vi "HandleCoincidenceData.vi"(4 "Added time":refnum<vi>, 6 "Seconds indicator":refnum<vi>, 7 "hit charts refnum cluster":T2, 8 "error in (no error)":errorcluster, 9 "coinc table":refnum<vi>, 10 "Seconds between updates":i32, 11 "Cluster":T3) -> (0 "error out":errorcluster)   [LabVIEW 2016]
uses:
  Typedefs/Coincidence histogram cluster refnum.ctl
  Typedefs/Hit chart cluster refnum.ctl
  Typedefs/Primary channel coincidence hunt.ctl
  Typedefs/Coincidence.ctl
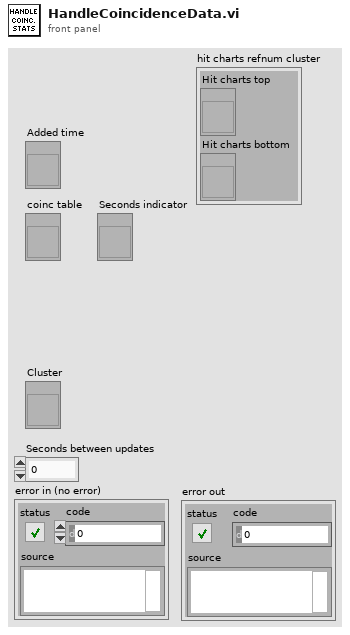
[diagram p1: front panel]
types:
  T1 = typedef "Hit chart cluster refnum.ctl" = refnum<vi>
  T2 = cluster{"Hit charts top":T1, "Hit charts bottom":T1}
  T3 = typedef "Coincidence histogram cluster refnum.ctl" = refnum<vi>
  T4 = typedef "Coincidence.ctl" = cluster{"Primary ID":i8, "Muon hit time":u64, "Secondary ID":i8, "DeltaT":i32}
  T5 = cluster{"Simultaneus muon tracks":cluster{"Top coinc":T4, "Bottom coinc":T4}[]}[]
  T6 = typedef "Primary channel coincidence hunt.ctl" = cluster{"Coincidences":T4[], "Secondary hits sorted":cluster{"ID":i8, "Non-coinc":u64[], "Coinc":u64[]}[], "Primary hits sorted":cluster{"ID":i8, "Non-coinc":u64[], "Coinc":u64[]}[]}
  T7 = cluster{"ID":i8, "Non-coinc":u64[], "Coinc":u64[]}[]
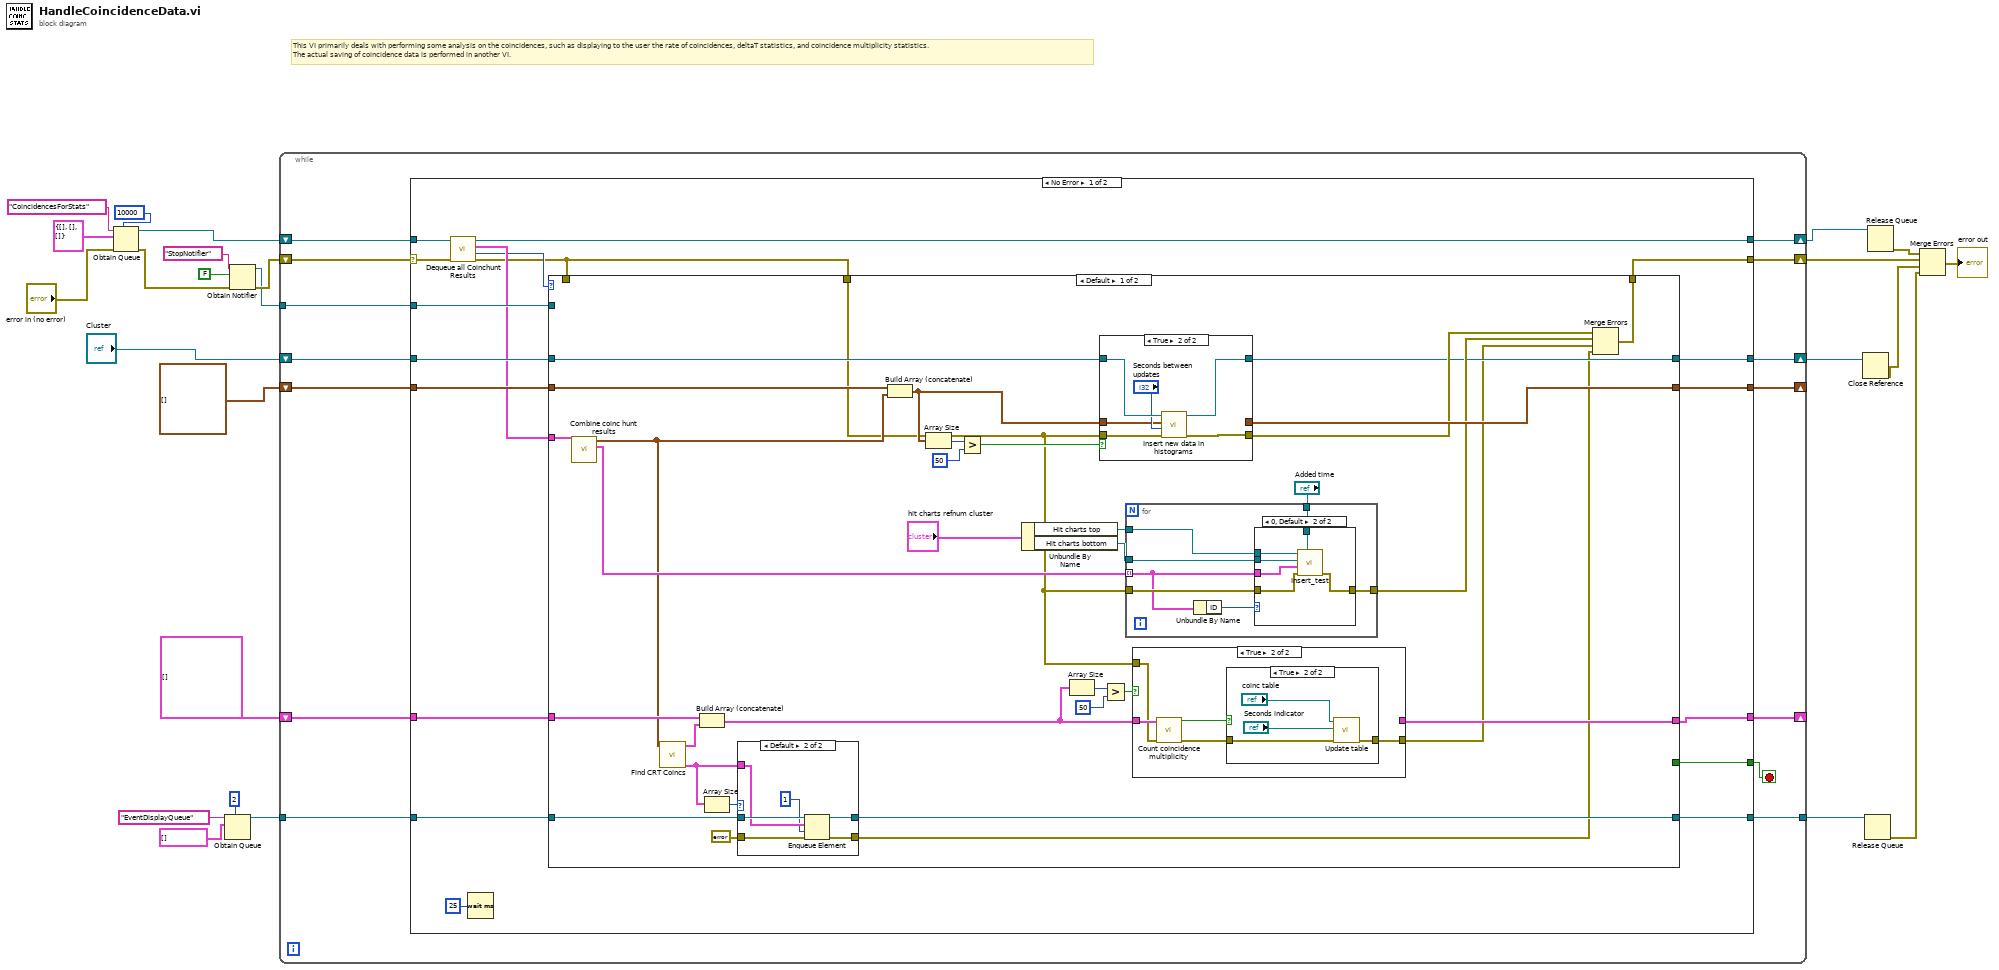
[diagram p0: block diagram]
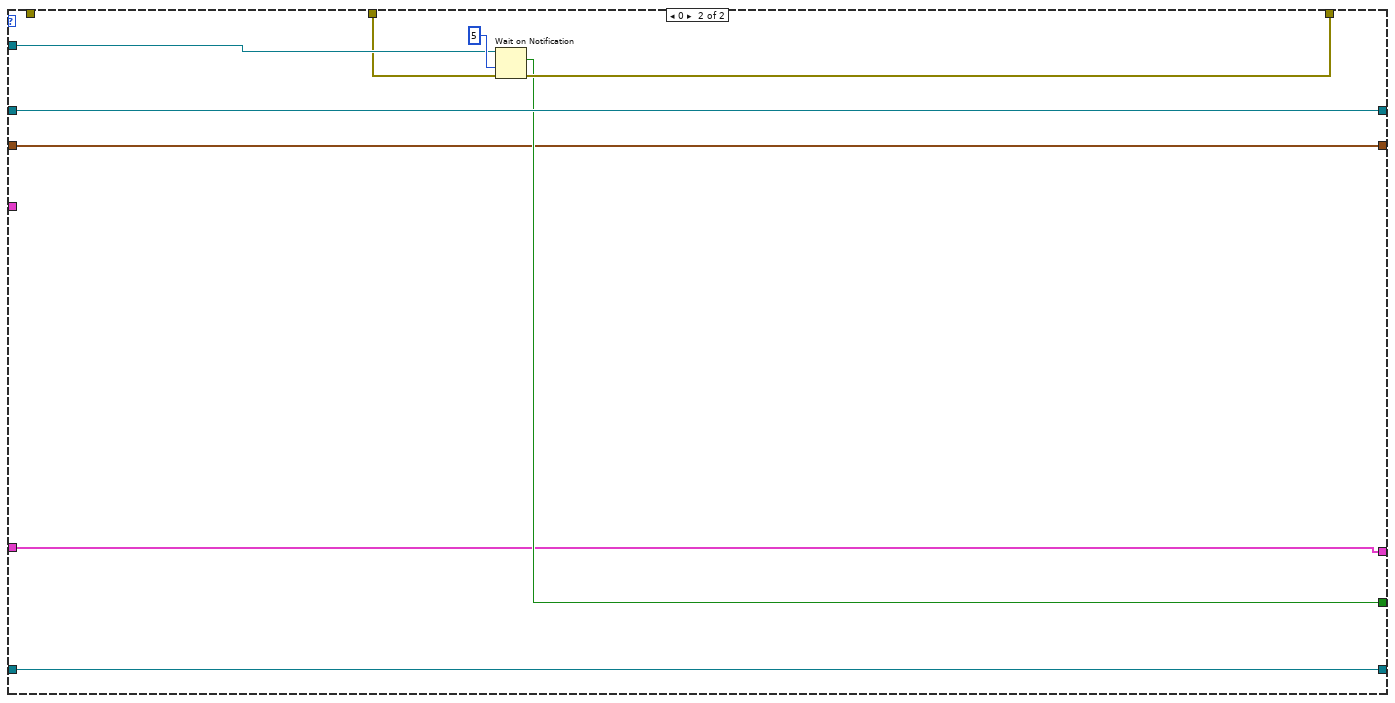
[diagram p7: hidden frame]
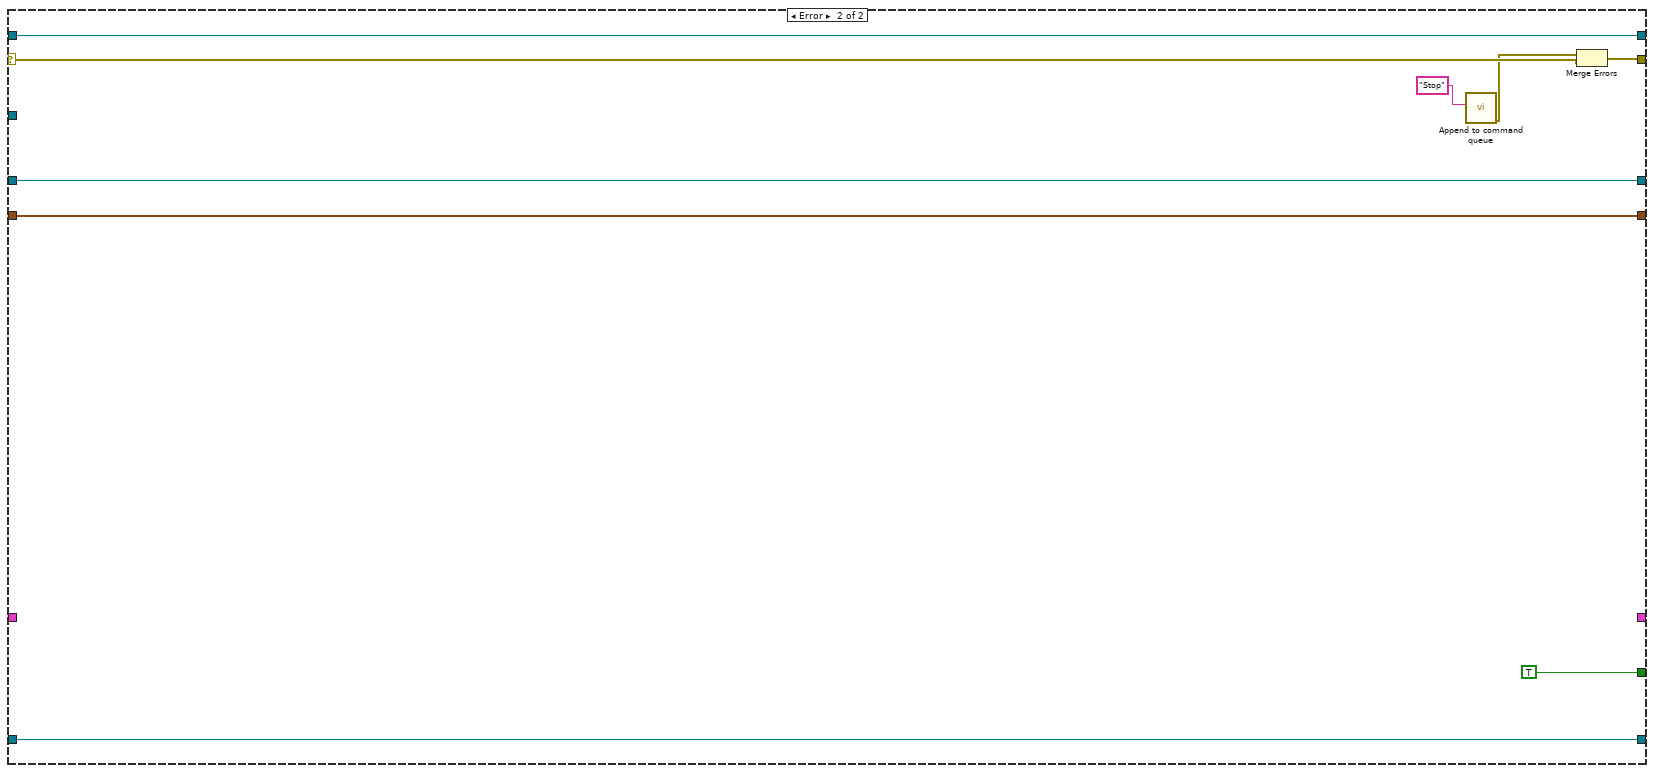
[diagram p8: hidden frame]
diagram:
  # "This VI primarily deals with performing some analysis on the coincidences, such as displaying to the user the rate of coincidences, deltaT statistics, and coincidence multiplicity statistics.\nThe actual saving of coincidence data is performed in another VI."
  n1 = Obtain Queue(max queue size (-1, unlimited)=10000, name (unnamed)="CoincidencesForStats", element data type=T6 {"Coincidences"=[], "Secondary hits sorted"=[], "Primary hits sorted"=[]} ("Planar coincidence hunt result"), error in (no error)="error in (no error)") -> (queue out=w24:refnum<queue>, error out=w17:errorcluster)  [unwired: 1 in, 1 out]
  n2 = Obtain Queue(max queue size (-1, unlimited)=2, name (unnamed)="EventDisplayQueue", element data type=T5 [] ("Good tracks")) -> (queue out=w4:refnum<queue>)  [unwired: 2 in, 2 out]
  n3 = Obtain Notifier(name (unnamed)="StopNotifier", notification data type=FALSE, error in (no error)=w17) -> (notifier out=w15:refnum<notifier>, error out=w16:errorcluster)  [unwired: 1 in, 1 out]
  n4 = while {
    shift-right: [w37] -> w14
    shift-left: w16 -> [w33]
    shift-right: [w38] -> w25
    shift-left: w24 -> [w39]
    shift-right: [w36] -> w11
    shift-left: "Cluster" -> [w32]
    tunnel: w15 -> [w34]
    shift-right: [w30] -> _
    shift-left: T4[] [] ("Coincidences") -> [w31]
    shift-right: [w28] -> _
    shift-left: cluster{"CRT-wide coincs":T4[]}[] [] ("CRT-wide coincidences") -> [w29]
    tunnel: w4 -> [w27]
    tunnel: [w26] -> w3
    stop <- w35 stop-if-true
    n5 = case shown="No Error" w33 {
      selector: w33 -> [w49 w150]
      tunnel: w39 -> [w50 w146]
      tunnel: [w48 w146] -> w38
      tunnel: [w57 w148] -> w37
      tunnel: w32 -> [w53 w145]
      tunnel: [w56 w145] -> w36
      tunnel: [w55 TRUE] -> w35
      tunnel: w34 -> [w54 _]
      tunnel: w31 -> [w52 w144]
      tunnel: [w51 w144] -> w30
      tunnel: w29 -> [w44 _]
      tunnel: [w43 _] -> w28
      tunnel: w27 -> [w42 w143]
      tunnel: [w41 w143] -> w26
      frame No Error {
        n6 = call "Dequeue all Coinchunt Results.vi"("error in (no error)"=w49, "Queue in"=w50) -> ("error out"=w40:errorcluster, "elements dequeued"=w46:i32, "Dequeued elements"=w47:T6[], "Queue out"=w48:refnum<queue>)  [unwired: 6 in]
        n7 = Wait (ms)(milliseconds to wait=u32 25) -> ()  [unwired: 1 out]
        n8 = case shown="Default" w46 {
          tunnel: w47 -> [w83 _]
          tunnel: [w79 w139] -> w57
          tunnel: w53 -> [w90 w142]
          tunnel: [w78 w142] -> w56
          tunnel: w54 -> [_ w140]
          tunnel: [_ w138] -> w55
          tunnel: w52 -> [w81 w137]
          tunnel: [w86 w137] -> w51
          tunnel: w40 -> [w63 w136]
          tunnel: w44 -> [w76 w135]
          tunnel: [w70 w135] -> w43
          tunnel: w42 -> [w68 w134]
          tunnel: [w67 w134] -> w41
          tunnel: w40 -> [_ _]
          frame Default {
            n9 = call "Combine coinc hunt results.vi"("Dequeued elements"=w83) -> ("Combined hits"=w77:T7, "Coincidences"=w69:T4[])  [unwired: 9 in]
            n10 = call "Find CRT Coincs.vi"("Coincidences"=w69) -> ("Good tracks"=w66:T5, "CRT-wide coincidences"=w75:cluster{"CRT-wide coincs":T4[]}[])  [unwired: 8 in, 1 out]
            n11 = Build Array (concatenate)(w76, w75) -> (w72:cluster{"CRT-wide coincs":T4[]}[])
            n12 = Array Size(array=w66) -> (size(s)=w65:i32)
            n13 = case shown="Default" w65 {
              tunnel: w68 -> [w92 w98]
              tunnel: [w92 w97] -> w67
              tunnel: w66 -> [_ w96]
              tunnel: [w91 w94] -> w62
              tunnel: errorcluster {"status"=FALSE, "code"=0, "source"=""} ("error out") -> [w91 w93]
              frame 0 {
              }
              frame Default {
                n14 = Enqueue Element(queue=w98, element=w96, timeout in ms (-1)=1, error in (no error)=w93) -> (queue out=w97:refnum<queue>, error out=w94:errorcluster)  [unwired: 1 out]
              }
            }
            n15 = Build Array (concatenate)(w81, w69) -> (w82:T4[])
            n16 = Array Size(array=w82) -> (size(s)=w89:i32)
            n17 = Greater?(x=w89, y=50) -> (0:w87:bool)
            n18 = Unbundle By Name("hit charts refnum cluster") -> ("Hit charts top"=w59:T1, "Hit charts bottom"=w58:T1)
            n19 = Array Size(array=w72) -> (size(s)=w73:i32)
            n20 = case shown="True" w87 {
              tunnel: w90 -> [w112 w119]
              tunnel: [w112 w118] -> w78
              tunnel: w82 -> [w113 w115]
              tunnel: [w113 _] -> w86
              tunnel: w63 -> [w111 w117]
              tunnel: [w111 w114] -> w85
              frame False {
              }
              frame True {
                n21 = call "Insert new data in histograms.vi"("Error in"=w117, "Seconds between updates"="Seconds between updates", "Coincidences"=w115, "Cluster"=w119) -> ("error out"=w114:errorcluster, "Cluster"=w118:T3)  [unwired: 6 in]
              }
            }
            n22 = Greater?(x=w73, y=50) -> (0:w71:bool)
            n23 = for {
              tunnel: w77 -> [w123] mode=indexing
              tunnel: w63 -> [w126]
              tunnel: [w125] -> w84
              tunnel: "Added time" -> [w124]
              tunnel: w59 -> [w121]
              tunnel: w58 -> [w120]
              n24 = Unbundle By Name(w123) -> ("ID"=w122:i8)
              n25 = case shown="0, Default" w122 {
                tunnel: w123 -> [_ w133]
                tunnel: w126 -> [w127 w132]
                tunnel: w121 -> [_ w131]
                tunnel: w120 -> [_ w130]
                tunnel: [w127 w129] -> w125
                tunnel: w124 -> [_ w128]
                frame 99 {
                }
                frame 0, Default {
                  n26 = call "Insert_test.vi"("Added time"=w128, "error in (no error)"=w132, "Sorted hits"=w133, "Bottom hit charts"=w130, "Top hit charts"=w131) -> ("error out"=w129:errorcluster)  [unwired: 6 in]
                }
              }
            }
            n27 = case shown="True" w71 {
              tunnel: w72 -> [w100 w105]
              tunnel: [w100 _] -> w70
              tunnel: [w99 w103] -> w64
              tunnel: w63 -> [w99 w101]
              frame False {
              }
              frame True {
                n28 = call "Count coincidence multiplicity.vi"("error in"=w101, "CRT-wide coincidences"=w105) -> ("error out"=w102:errorcluster, "New data?"=w104:bool)  [unwired: 8 in]
                n29 = case shown="True" w104 {
                  tunnel: w102 -> [w106 w110]
                  tunnel: [w106 w109] -> w103
                  frame False {
                  }
                  frame True {
                    n30 = call "Update table.vi"("error in"=w110, "Seconds indicator"="Seconds indicator", "Table"="coinc table") -> ("error out"=w109:errorcluster)  [unwired: 8 in]
                  }
                }
              }
            }
            n31 = Merge Errors(w85, w84, w64, w62) -> (w79:errorcluster)
          }
          frame 0 {
            n32 = Wait on Notification(notifier=w140, timeout in ms (-1)=5, error in (no error)=w136) -> (notification=w138:bool, error out=w139:errorcluster)  [unwired: 1 in, 2 out]
          }
        }
      }
      frame Error {
        n33 = call "Append to command queue.vi"("Single command"="Stop") -> ("error out"=w149:errorcluster)  [unwired: 10 in]
        n34 = Merge Errors(w149, w150) -> (w148:errorcluster)
      }
    }
  }
  n35 = Close Reference(reference=w11) -> (error out=w10:errorcluster)  [unwired: 1 in]
  n36 = Release Queue(queue=w3) -> (error out=w2:errorcluster)  [unwired: 2 in, 2 out]
  n37 = Release Queue(queue=w25) -> (error out=w13:errorcluster)  [unwired: 2 in, 2 out]
  n38 = Merge Errors(w13, w14, w10, w2) -> (→"error out":errorcluster)
